vi "LV2010_rshmc804x_SimpleExample.vi"() -> ()   [LabVIEW 2016]
uses:
  <instrlib>/Rohde&Schwarz HMC 804x Power Supplies/Rohde&Schwarz HMC 804x Power Supplies.lvlib
panel:
  out "Screenshot":picture
  in  "CH2 Current":dbl=2.2
  in  "CH1 Current":dbl=1.1
  in  "CH1 enabled":bool caption="CH1 ON"
  in  "CH2 enabled":bool caption="CH2 ON"
  in  "CH2 Voltage":dbl=5.0
  in  "CH1 Voltage":dbl=3.0
  # "HMC804x simple example"
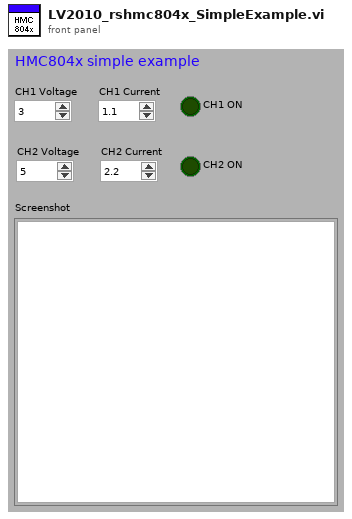
[diagram p1: front panel]
types:
  T1 = typedef "imagedata.ctl" = cluster{"image type":i32, "image depth":i32, "image":u8[], "mask":u8[], "colors":u32[], "Rectangle":cluster{"left":i16, "top":i16, "right":i16, "bottom":i16}}
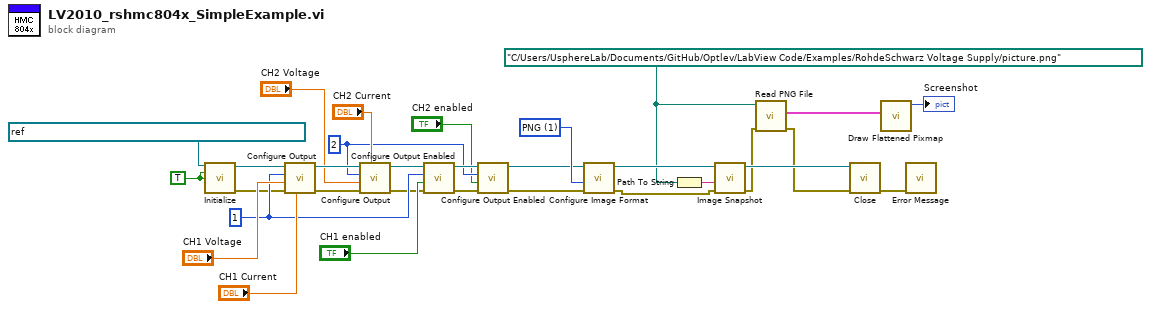
[diagram p0: block diagram]
diagram:
  w12 = path "C:/Users/UsphereLab/Documents/GitHub/Optlev/LabView Code/Examples/RohdeSchwarz Voltage Supply/picture.png" ("path to BMP file")
  w14 = 1 items=["BMP", "PNG"] ("Image Format (BMP)")
  w19 = TRUE ("ID Query (T: Check)")
  w22 = 2 ("Channel (1)")
  w24 = 1 ("Channel (1)")
  n1 = call <instrlib>:"Initialize.vi"("VISA resource name"=refnum<visa-resource-name> "USB0::0x0AAD::0x0197::5601.1414k02-100769::INSTR", "ID Query (T: Check)"=w19, "Reset (T: Reset)"=w19) -> ("VISA resource name out"=w28:refnum<visa-resource-name>, "error out"=w9:errorcluster)  [unwired: 11 in]
  n2 = call <instrlib>:"Configure Output.vi"("Current (0.0)"="CH1 Current", "error in (no error)"=w9, "Voltage (0.0)"="CH1 Voltage", "Channel (1)"=w24, "VISA resource name"=w28) -> ("error out"=w8:errorcluster, "VISA resource name out"=w27:refnum<visa-resource-name>)  [unwired: 5 in]
  n3 = call <instrlib>:"Configure Output.vi"("Current (0.0)"="CH2 Current", "error in (no error)"=w8, "Voltage (0.0)"="CH2 Voltage", "Channel (1)"=w22, "VISA resource name"=w27) -> ("error out"=w7:errorcluster, "VISA resource name out"=w25:refnum<visa-resource-name>)  [unwired: 5 in]
  n4 = call <instrlib>:"Configure Output Enabled.vi"("error in (no error)"=w7, "Enabled (Off)"="CH1 enabled", "Channel (1)"=w24, "VISA resource name"=w25) -> ("error out"=w6:errorcluster, "VISA resource name out"=w23:refnum<visa-resource-name>)  [unwired: 6 in]
  n5 = call <instrlib>:"Configure Output Enabled.vi"("error in (no error)"=w6, "Enabled (Off)"="CH2 enabled", "Channel (1)"=w22, "VISA resource name"=w23) -> ("error out"=w5:errorcluster, "VISA resource name out"=w11:refnum<visa-resource-name>)  [unwired: 6 in]
  n6 = call <instrlib>:"Configure Image Format.vi"("error in (no error)"=w5, "Image Format (BMP)"=w14, "VISA resource name"=w11) -> ("error out"=w4:errorcluster, "VISA resource name out"=w15:refnum<visa-resource-name>)  [unwired: 7 in]
  n7 = Path To String(path=w12) -> (string=w13:string)
  n8 = call <instrlib>:"Image Snapshot.vi"("error in (no error)"=w4, "Destination (\"\")"=w13, "VISA resource name"=w15) -> ("error out"=w3:errorcluster, "VISA resource name out"=w16:refnum<visa-resource-name>)  [unwired: 7 in]
  n9 = call <vilib>:"Read PNG File.vi"("error in (no error)"=w3, "path to PNG file"=w12) -> ("error out"=w2:errorcluster, "image data"=w18:T1)  [unwired: 7 in, 1 out]
  n10 = call <instrlib>:"Close.vi"("error in (no error)"=w2, "VISA resource name"=w16) -> ("error out"=w1:errorcluster)  [unwired: 9 in]
  n11 = call <vilib>:"Draw Flattened Pixmap.vi"("image data"=w18) -> ("new picture"=→"Screenshot":picture)  [unwired: 8 in]
  n12 = call <instrlib>:"Error Message.vi"("error in (no error)"=w1) -> ()  [unwired: 10 in, 5 out]
